vi "Shutdown.vi"(8 "error in (no error)":errorcluster, 11 "GIS Printer in":refnum<class "GIS Printer.lvclass">) -> (0 "error out":errorcluster, 3 "GIS Printer out":refnum<class "GIS Printer.lvclass">)   [LabVIEW 2022 SP3, in "GIS Printer.lvclass"]
uses:
  GIS Printer.lvclass
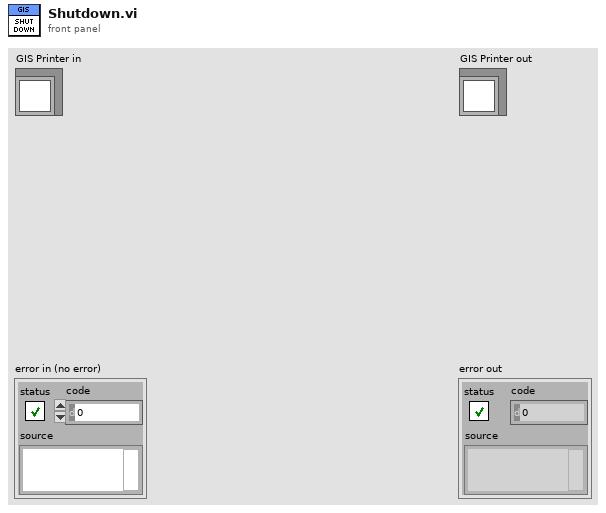
[diagram p1: front panel]
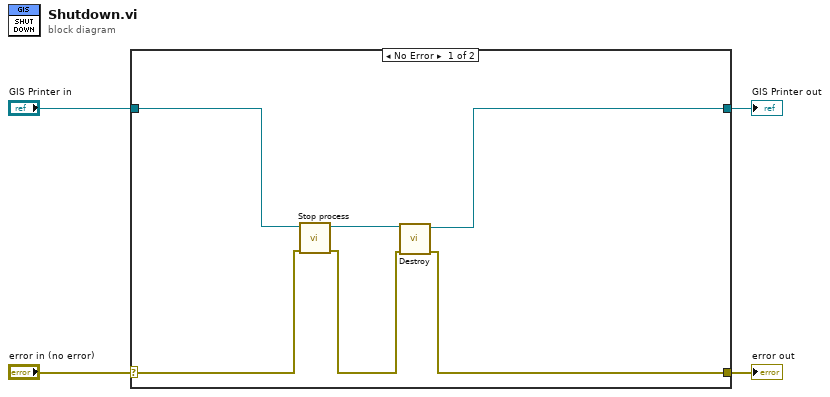
[diagram p0: block diagram]
diagram:
  n1 = case shown="No Error" "error in (no error)" {
    selector: "error in (no error)" -> [w10 w12]
    tunnel: [w7 w12] -> w3
    tunnel: [w6 w11] -> w1
    tunnel: "GIS Printer in" -> [w5 w11]
    frame No Error {
      n2 = call "Stop process.vi"("error in (no error)"=w10, "GIS Printer in"=w5) -> ("error out"=w8:errorcluster, "GIS Printer out"=w9:refnum<class "GIS Printer.lvclass">)  [unwired: 8 in]
      n3 = call-dynamic "Destroy.vi"("error in (no error)"=w8, "TopLevel in"=w9) -> ("error out"=w7:errorcluster, "TopLevel out"=w6:refnum<class "GIS Printer.lvclass">)  [unwired: 8 in]
    }
    frame Error {
    }
  }
  "error out" <- w3
  "GIS Printer out" <- w1
